vi "Fire Alarm System - Select.vi"() -> ()   [LabVIEW 2021]
uses:
  <vilib>/MakerHub/LINX/Public/Peripherals/Analog/Analog Read 1 Chan.vi
  <vilib>/MakerHub/LINX/Public/Peripherals/Digital/Digital Write 1 Chan.vi
  <vilib>/MakerHub/LINX/Public/Peripherals/Digital/Digital Read 1 Chan.vi
  <vilib>/MakerHub/LINX/Public/Peripherals/PWM/PWM Set Duty Cycle 1 Chan.vi
  <vilib>/MakerHub/LINX/Public/Peripherals/Analog/Analog Read N Chans.vi
  <vilib>/MakerHub/LINX/Public/Peripherals/Digital/Digital Write N Chans.vi
  <vilib>/MakerHub/LINX/Public/Peripherals/Digital/Digital Read N Chans.vi
  <vilib>/MakerHub/LINX/Private/Local IO/LinxAnalogRead.vi
  <vilib>/MakerHub/LINX/Public/Utilities/Check Channel.vi
  <vilib>/MakerHub/LINX/Private/Local IO/LinxDigitalWrite.vi
  <vilib>/MakerHub/LINX/Private/Local IO/LinxDigitalRead.vi
  <vilib>/MakerHub/LINX/Public/Utilities/Open Serial.vi
  <vilib>/MakerHub/LINX/Private/Utilties/Generate Error.vi
  <vilib>/MakerHub/LINX/Public/Sensors/Temperature/TMP3x/TMP35.vi
  <vilib>/MakerHub/LINX/Public/Peripherals/PWM/PWM Set Duty Cycle N Chans.vi
  <vilib>/MakerHub/LINX/LMH-LINX.lvlib
  <vilib>/MakerHub/LINX/Public/Sensors/Temperature/TMP3x/TMP3x.lvlib
panel:
  out "?":bool
  in  "Buzzer":u8
  in  "Punp":bool
  in  "DO Channel 5":u8
  in  "Motor Speed 2":dbl(knob) scale=0.0..1.0
  in  "PWM Channel 2":u8
  in  "CW":bool
  in  "DO Channel 4":u8
  in  "DO Channel 3":u8
  in  "Motor Speed":dbl(knob) scale=0.0..1.0
  in  "PWM Channel":u8
  out "Error Out":errorcluster
  out "Waveform Chart":dbl(graph)
  out "Meter":dbl(knob) scale=0.0..10.0
  in  "Analog Channel 3":u8
  out "Fire":bool
  in  "DO Channel 2":u8
  in  "DI Channel":u8
  out "Temperature":u8(slide) scale=0.0..50.0
  in  "Temperature A. Channel":u8
  out "Temp C":dbl format="%#.1g"
  in  "stop":bool
  in  "Smoke LED DO Channel":u8
  out "Smoke":bool
  in  "Serial Port":refnum<visa-resource-name>="N/A"
  in  "Smoke Reference Value":dbl
  out "Smoke o/p":dbl
  in  "Smoke Sensor A.\n Channel":u8
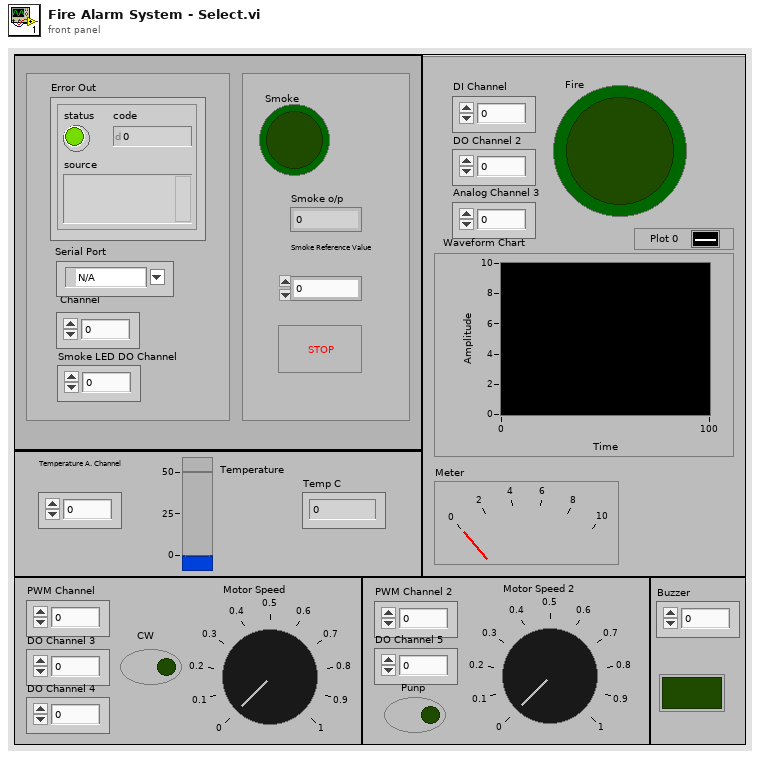
[diagram p1: front panel]
types:
  T1 = typedef "LMH-LINX.lvlib/LINX Ref.ctl" = cluster{"IO":T2, "Interface":T3, "LINX Device Config":T4}
  T2 = typedef "LMH-LINX.lvlib/Platform.ctl" = enum16{"Remote", "Local"}
  T3 = typedef "LMH-LINX.lvlib/Interface.ctl" = enum16{"Serial", "TCP"}
  T4 = typedef "LMH-LINX.lvlib/Device.lvlib/LINX Device Config.ctl" = cluster{"Interface":T3, "COM Port":refnum<visa-resource-name>, "TCP Configuration":T5, "Device Family":u8, "Device ID":u8, "Device Name":string, "TCP Ref":refnum<k5>, "Channels":T6}
  T5 = typedef "LMH-LINX.lvlib/Device.lvlib/TCP Config.ctl" = cluster{"IP Address":string, "Port":u16}
  T6 = typedef "LMH-LINX.lvlib/Channels.ctl" = cluster{"DI":u8[], "DO":u8[], "AI":u8[], "AO":u8[], "PWM":u8[], "QE":u8[], "UART":u8[], "I2C 2":u8[], "SPI":u8[], "CAN":u8[], "Servo":u8[], "AI Ref (V)":dbl, "AI Resolution (Bits)":u8, "AO Ref (V)":dbl, "AO Resolution (Bits)":u8}
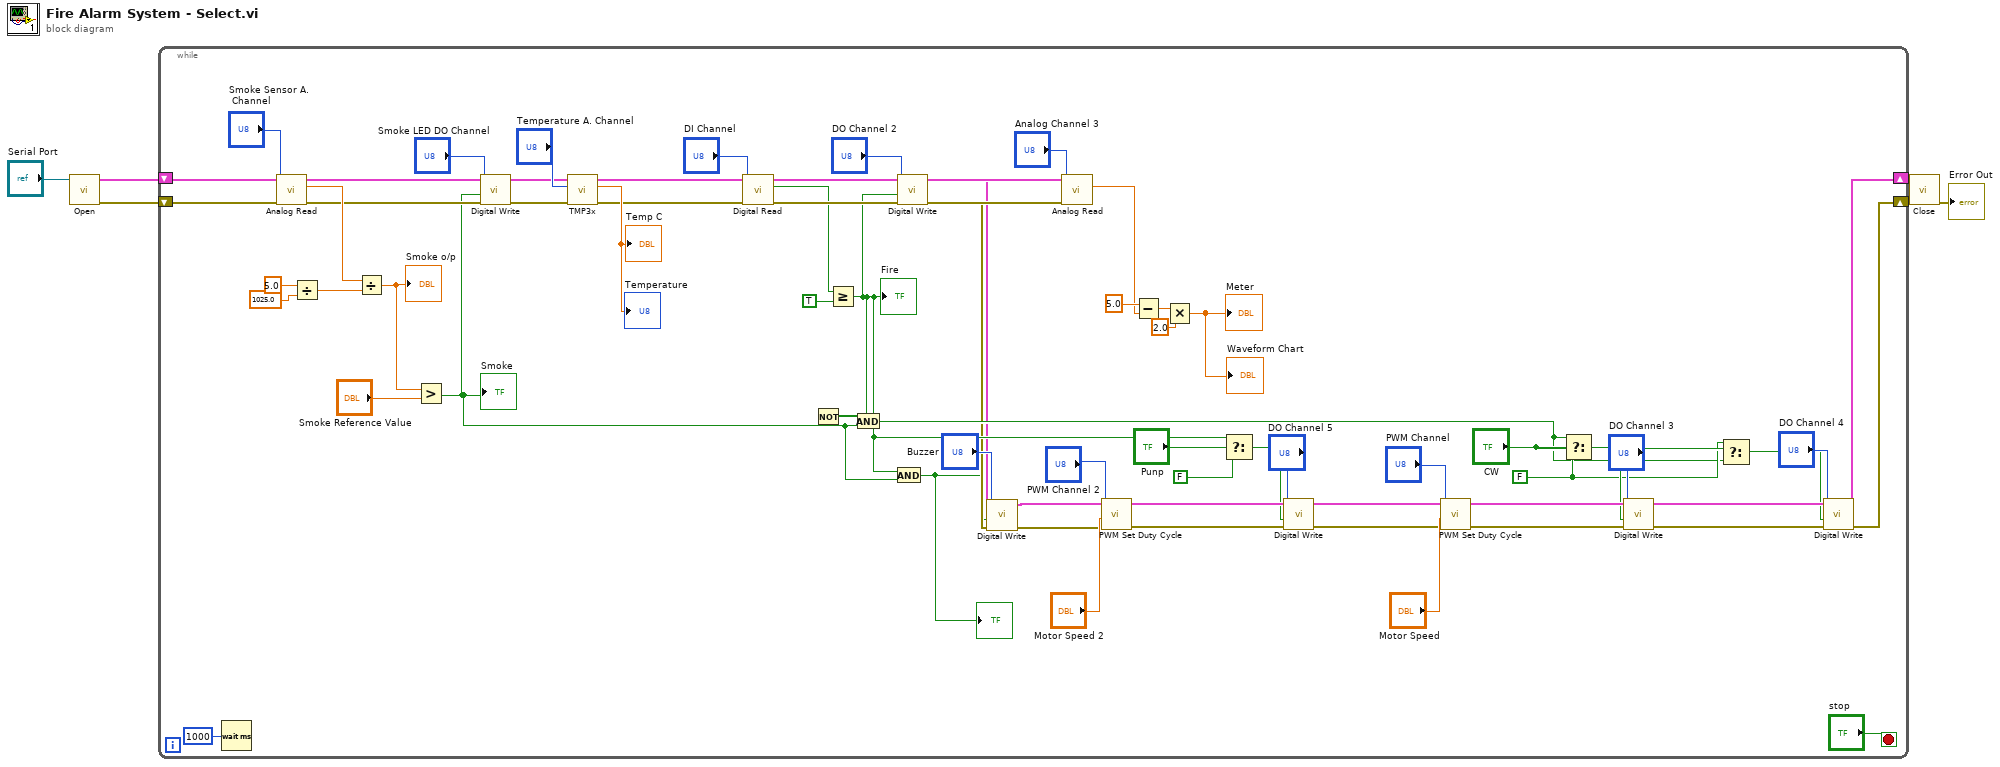
[diagram p0: block diagram]
diagram:
  n1 = call-poly <vilib>:"Open.vi"("Serial Port"="Serial Port") -> ("Error Out"=w5:errorcluster, "LINX Resource"=w4:T1)  [unwired: 8 in, 1 out]
  n2 = while {
    shift-right: [w30] -> w2
    shift-left: w5 -> [w41]
    shift-right: [w31] -> w3
    shift-left: w4 -> [w42]
    stop <- "stop" stop-if-true
    w27 = FALSE ("f")
    n3 = Wait (ms)(milliseconds to wait=u32 1000) -> ()  [unwired: 1 out]
    n4 = call-poly <vilib>:"Analog Read.vi"("Error In"=w41, "Analog Channel"="Smoke Sensor A.\n Channel", "LINX Resource"=w42) -> ("Error Out"=w67:errorcluster, "Voltage"=w72:dbl, "LINX Resource"=w68:T1)  [unwired: 5 in, 1 out]
    n5 = Divide(x=5.0, y=1025.0) -> (x/y=w73:dbl)
    n6 = Divide(x=w72, y=w73) -> (x/y=w63:dbl)
    "Smoke o/p" <- w63
    n7 = Greater?(x=w63, y="Smoke Reference Value") -> (0:w15:bool)
    "Smoke" <- w15
    n8 = call-poly <vilib>:"Digital Write.vi"("Error In"=w67, "Output Value"=w15, "DO Channel"="Smoke LED DO Channel", "LINX Resource"=w68) -> ("Error Out"=w60:errorcluster, "LINX Resource"=w61:T1)  [unwired: 6 in]
    n9 = call-poly <vilib>:"TMP3x.vi"("Error In"=w60, "Analog Channel"="Temperature A. Channel", "LINX Resource"=w61) -> ("Error Out"=w46:errorcluster, "Temp C"=→"Temp C" →"Temperature":dbl, "LINX Resource"=w47:T1)  [unwired: 6 in]
    n10 = call-poly <vilib>:"Digital Read.vi"("Error In"=w46, "DI Channel"="DI Channel", "LINX Resource"=w47) -> ("Error Out"=w57:errorcluster, "DI Value"=w49:bool, "LINX Resource"=w58:T1)  [unwired: 6 in]
    n11 = Greater Or Equal?(x=w49, y=TRUE) -> (x >= y?=w14:bool)
    "Fire" <- w14
    n12 = Not(x=w14) -> (.not. x?=w38:bool)
    n13 = And(x=w38, y=w15) -> (x .and. y?=w26:bool)
    n14 = And(x=w14, y=w15) -> (x .and. y?=w7:bool)
    "?" <- w7
    n15 = call-poly <vilib>:"Digital Write.vi"("Error In"=w57, "Output Value"=w14, "DO Channel"="DO Channel 2", "LINX Resource"=w58) -> ("Error Out"=w53:errorcluster, "LINX Resource"=w54:T1)  [unwired: 6 in]
    n16 = call-poly <vilib>:"Analog Read.vi"("Error In"=w53, "Analog Channel"="Analog Channel 3", "LINX Resource"=w54) -> ("Error Out"=w12:errorcluster, "Voltage"=w50:dbl, "LINX Resource"=w11:T1)  [unwired: 5 in, 1 out]
    n17 = call-poly <vilib>:"Digital Write.vi"("Error In"=w12, "Output Value"=w7, "DO Channel"="Buzzer", "LINX Resource"=w11) -> ("Error Out"=w8:errorcluster, "LINX Resource"=w9:T1)  [unwired: 6 in]
    n18 = call-poly <vilib>:"PWM Set Duty Cycle.vi"("Error In"=w8, "Duty Cycle (0-1)"="Motor Speed 2", "PWM Channel"="PWM Channel 2", "LINX Resource"=w9) -> ("Error Out"=w21:errorcluster, "LINX Resource"=w22:T1)  [unwired: 6 in]
    n19 = Subtract(x=5.0, y=w50) -> (x-y=w45:dbl)
    n20 = Multiply(x=w45, y=2.0) -> (x*y=→"Meter" →"Waveform Chart":dbl)
    n21 = Select(t=w14, s="Punp", f=FALSE) -> (s? t:f=w20:bool)
    n22 = call-poly <vilib>:"Digital Write.vi"("Error In"=w21, "Output Value"=w20, "DO Channel"="DO Channel 5", "LINX Resource"=w22) -> ("Error Out"=w16:errorcluster, "LINX Resource"=w17:T1)  [unwired: 6 in]
    n23 = call-poly <vilib>:"PWM Set Duty Cycle.vi"("Error In"=w16, "Duty Cycle (0-1)"="Motor Speed", "PWM Channel"="PWM Channel", "LINX Resource"=w17) -> ("Error Out"=w35:errorcluster, "LINX Resource"=w36:T1)  [unwired: 6 in]
    n24 = Select(t=w26, s="CW", f=w27) -> (s? t:f=w29:bool)
    n25 = call-poly <vilib>:"Digital Write.vi"("Error In"=w35, "Output Value"=w29, "DO Channel"="DO Channel 3", "LINX Resource"=w36) -> ("Error Out"=w32:errorcluster, "LINX Resource"=w34:T1)  [unwired: 6 in]
    n26 = Select(t=w27, s="CW", f=w26) -> (s? t:f=w25:bool)
    n27 = call-poly <vilib>:"Digital Write.vi"("Error In"=w32, "Output Value"=w25, "DO Channel"="DO Channel 4", "LINX Resource"=w34) -> ("Error Out"=w30:errorcluster, "LINX Resource"=w31:T1)  [unwired: 6 in]
  }
  n28 = call <vilib>:"Close.vi"("Error In"=w2, "LINX Resource"=w3) -> ("Error Out"=→"Error Out":errorcluster)  [unwired: 9 in]
